vi "UpdateDeviceStatus.vi"(5 "error in":errorcluster) -> (20 "andor 1":bool, 22 "temperatureValuesOut[0]":i32, 23 "error out":errorcluster, 24 "andor 0":bool, 26 "temperatureValuesOut[1]":i32)   [LabVIEW 2011]
uses:
  Utilities/controls/ctlSeqFNs_Andor_temp.ctl
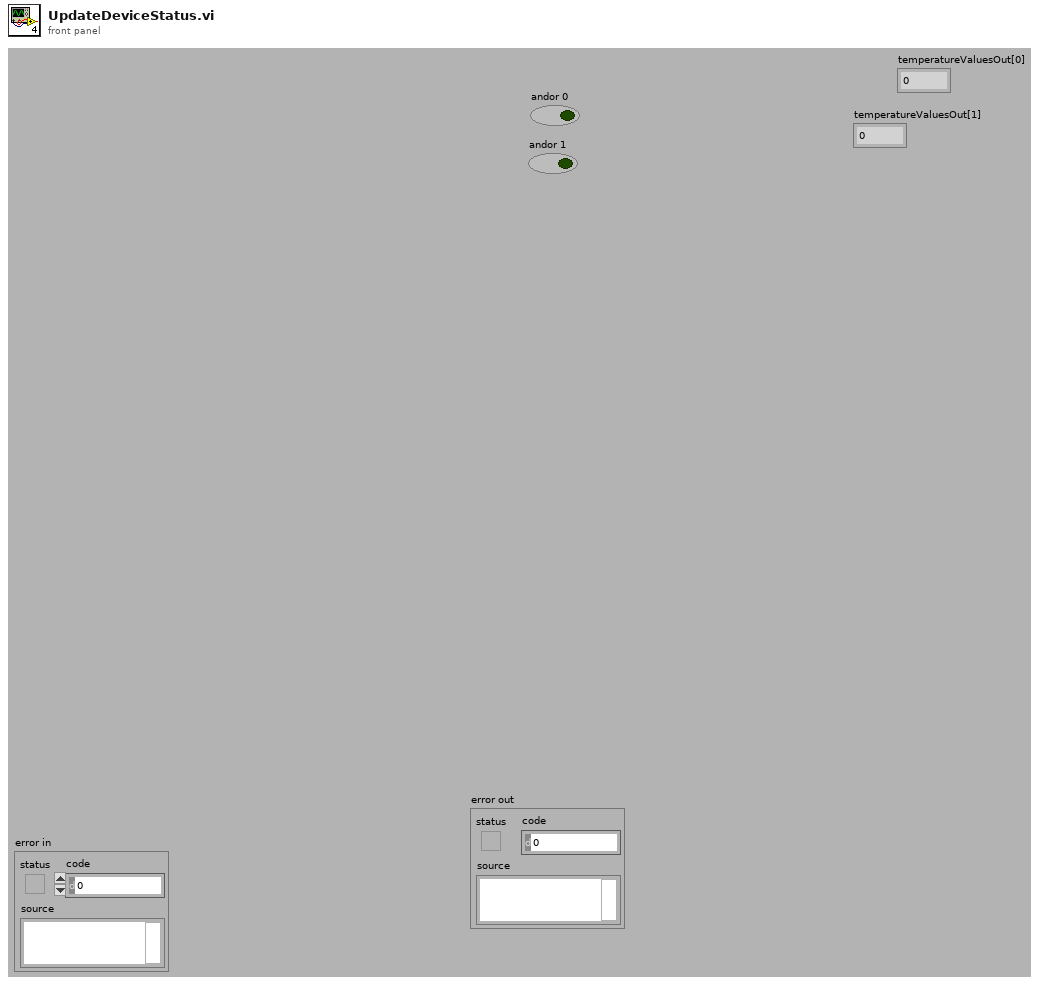
[diagram p1: front panel]
types:
  T1 = typedef "ctlSeqFNs_Andor_temp.ctl" = enum16{"Temperature  FALSE", "Temperature OK"}
  T2 = cluster{"temperatureValuesOut[0]":i32, "temperatureValuesOut[1]":i32, "temperatureValuesOut[2]":i32, "temperatureValuesOut[3]":i32, "temperatureValuesOut[4]":i32, "temperatureValuesOut[5]":i32, "temperatureValuesOut[6]":i32, "temperatureValuesOut[7]":i32, "temperatureValuesOut[8]":i32}
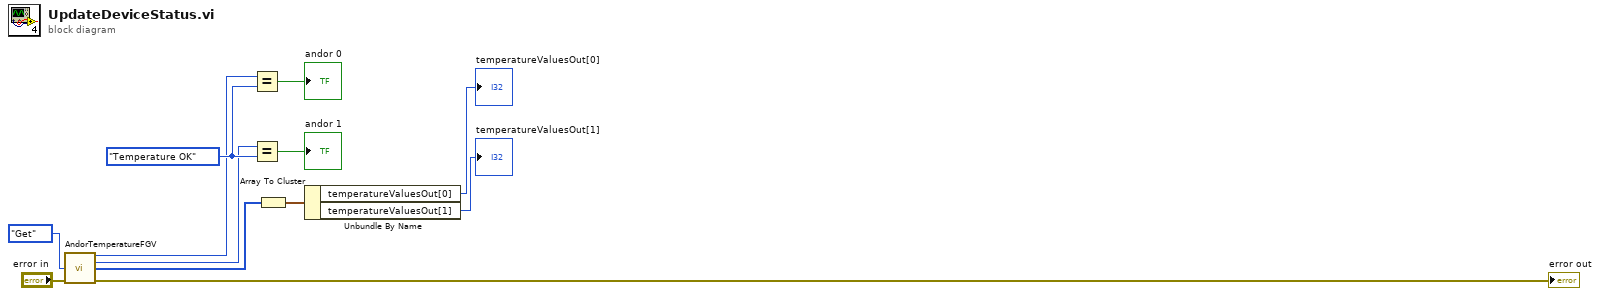
[diagram p0: block diagram]
diagram:
  w9 = ctlSeqFNs_Andor_temp."Temperature OK" ("TemperaturStatus")
  n1 = call "AndorTemperatureFGV.vi"("Set_Get"=enum16{"Set", "Get"}."Get", "error in"="error in") -> ("Andor 0 Temperature"=w7:T1, "Andor 1 Temperature"=w8:T1, "temperatureValuesOut"=w5:i32[], "error out"=→"error out":errorcluster)  [unwired: 10 in]
  n2 = Equal?(x=w7, y=w9) -> (x = y?=→"andor 0":bool)
  n3 = Equal?(x=w8, y=w9) -> (x = y?=→"andor 1":bool)
  n4 = Array To Cluster(array=w5) -> (cluster=w4:T2)
  n5 = Unbundle By Name(w4) -> ("temperatureValuesOut[0]"=→"temperatureValuesOut[0]":i32, "temperatureValuesOut[1]"=→"temperatureValuesOut[1]":i32)
